vi "Main.vi"() -> ()   [LabVIEW 2020, in "Main.lvclass"]
uses:
  Main/Main.lvclass
  Coffee Shop/Coffee Shop.lvclass
  <vilib>/Asteme/Triarc Framework/Process/Process.lvclass
  <vilib>/Asteme/Triarc Framework/Application/Application.lvclass
  C:/Program Files (x86)/National Instruments/LabVIEW 2020/vi.lib/Asteme/Triarc Framework/Application/Application.lvclass
  C:/Program Files (x86)/National Instruments/LabVIEW 2020/vi.lib/Asteme/Triarc Framework/Process/Process.lvclass
  C:/Program Files (x86)/National Instruments/LabVIEW 2020/vi.lib/Asteme/Triarc Framework/Base/Base.lvclass
  C:/Program Files (x86)/National Instruments/LabVIEW 2020/vi.lib/Asteme/Triarc Framework/Error Handler Interface/Error Handler Interface.lvclass
  C:/Program Files (x86)/National Instruments/LabVIEW 2020/vi.lib/Asteme/Triarc Framework/Logging/Logging.lvclass
  C:/Users/anton/Documents/GitHub/Triarc-Examples/Coffee Shop/Coffee Shop/Coffee Shop.lvclass
panel:
  in  "Remove Customer":bool
  in  "Stop Button":bool
  in  "Remove Barista":bool
  in  "Show Barista Info":bool
  in  "Add Barista":bool
  in  "Baristas":i32(listbox)
  in  "Remove Cashier":bool
  in  "Show Cashier Info":bool
  in  "Add Cashier":bool
  in  "Cashiers":i32(listbox)
  in  "Show Customer Info":bool
  in  "Add Customer":bool
  in  "Customers":i32(listbox)
  # "Click + to add a customer actor to the system.\nClick Place Order to choose items for the customer to order.\nCustomer will wait until all items ordered are ready, then exit."
  # "Cashiers process orders into individual drink jobs and forwards those jobs to baristas.\nClick + to add a cashier actor to the system.\nClick - to remove a cashier from the system."
  # "Baristas process drink jobs and notify customers of completed drinks.\nAdd more baristas to the system by clicking +.  Pending jobs will be assigned to the next available barista.\nClick - to remove a barista from the system."
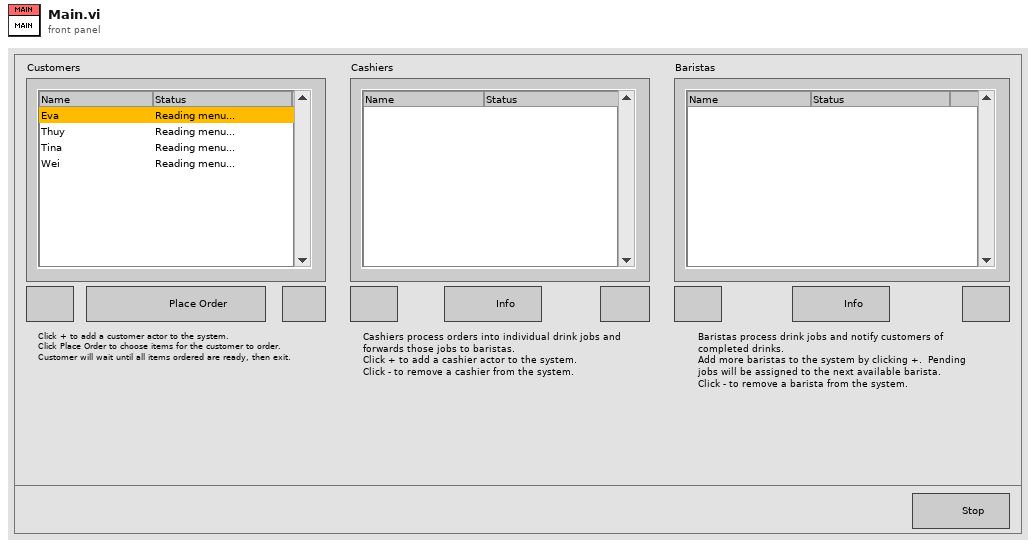
[diagram p1: front panel]
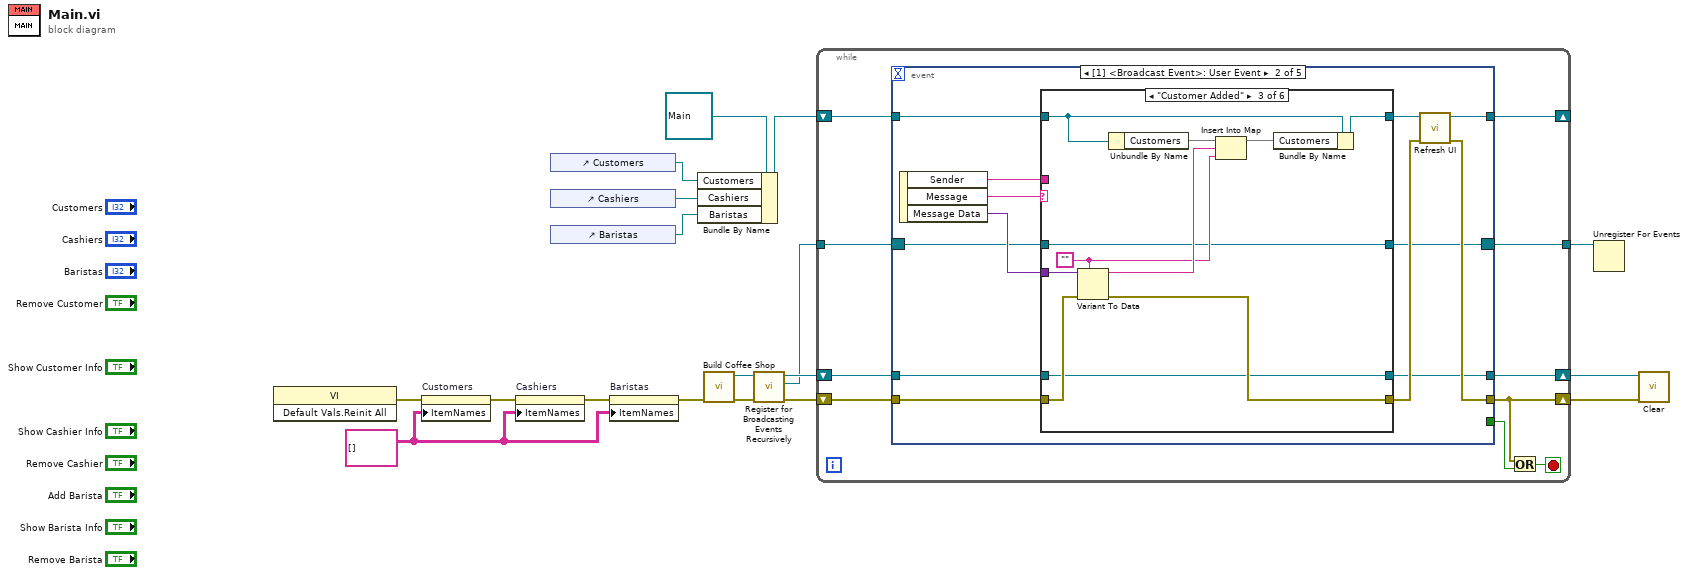
[diagram p0: block diagram]
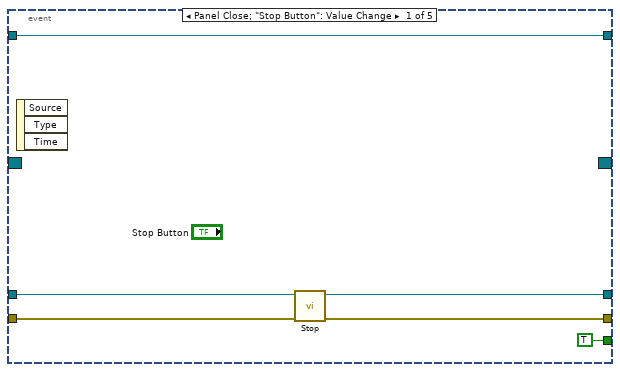
[diagram p2: hidden frame]
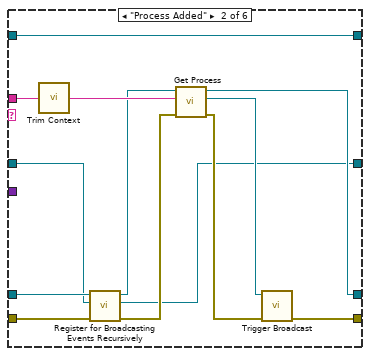
[diagram p4: hidden frame]
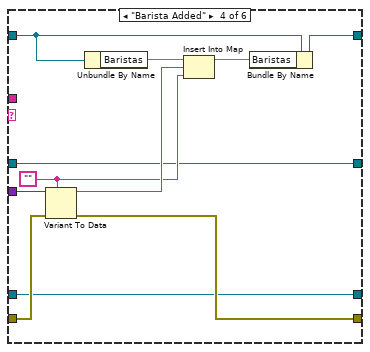
[diagram p5: hidden frame]
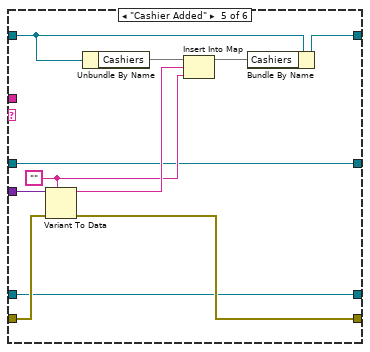
[diagram p6: hidden frame]
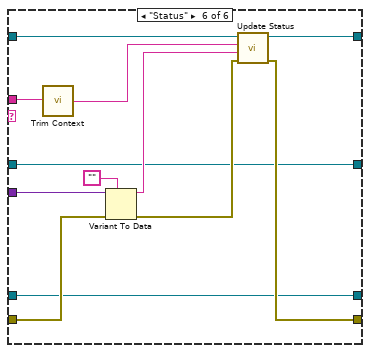
[diagram p7: hidden frame]
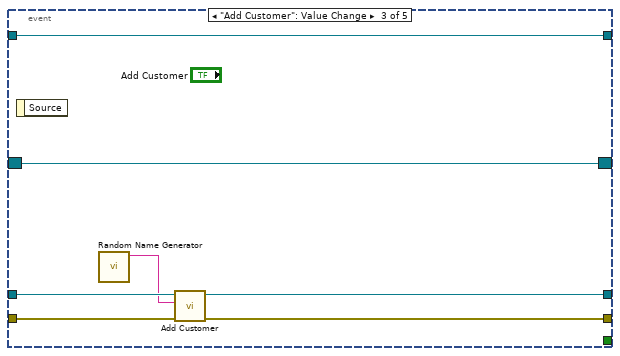
[diagram p8: hidden frame]
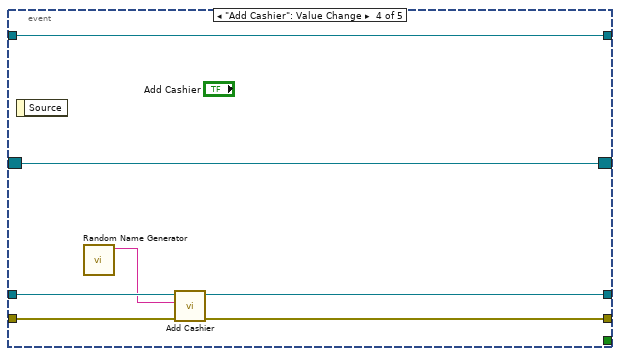
[diagram p9: hidden frame]
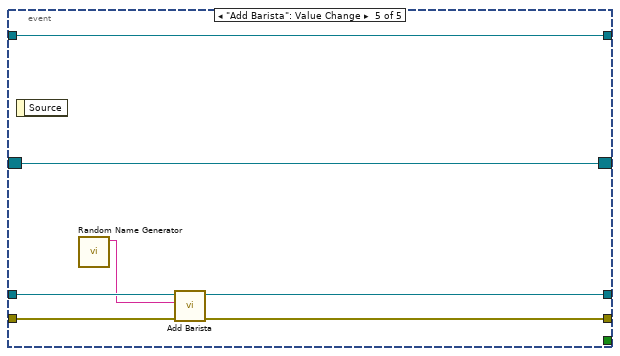
[diagram p10: hidden frame]
diagram:
  w11 = string[][] [] ("Item Names")
  n1 = invoke on="Invoke Node" class="VI" method="Default Vals.Reinit All"() -> (error out=w13:errorcluster)  [unwired: 3 in, 2 out]
  n2 = property on="Customers" class="MCListbox (strict)"(error in=w13, "ItemNames"=w11) -> (error out=w15:errorcluster)  [unwired: 1 in, 1 out]
  n3 = property on="Cashiers" class="MCListbox (strict)"(error in=w15, "ItemNames"=w11) -> (error out=w14:errorcluster)  [unwired: 1 in, 1 out]
  n4 = control-ref of="Customers"() -> (w8:refnum<vi>)
  n5 = control-ref of="Cashiers"() -> (w7:refnum<vi>)
  n6 = control-ref of="Baristas"() -> (w6:refnum<vi>)
  n7 = property on="Baristas" class="MCListbox (strict)"(error in=w14, "ItemNames"=w11) -> (error out=w12:errorcluster)  [unwired: 1 in, 1 out]
  n8 = Bundle By Name(cluster=refnum<class "Main.lvclass"> refnum ("Main.lvclass"), "Customers"=w8, "Cashiers"=w7, "Baristas"=w6) -> (w9:refnum<class "Main.lvclass">)
  n9 = call "Build Coffee Shop.vi"("error in (no error)"=w12) -> ("error out"=w4:errorcluster, "Coffee Shop Out"=w5:refnum<class "Coffee Shop.lvclass">)  [unwired: 9 in]
  n10 = call <vilib>:"Register for Broadcasting Events Recursively.vi"("error in (no error)"=w4, "Application In"=w5) -> ("error out"=w3:errorcluster, "Event Registration Refnum Out"=w1:refnum<event-registration>, "Application Out"=w2:refnum<class "Coffee Shop.lvclass">)  [unwired: 7 in]
  n11 = while {
    shift-right: [w27] -> w17
    shift-left: w3 -> [w28]
    shift-right: [w23] -> w16
    shift-left: w2 -> [w24]
    tunnel: w1 -> [w22]
    tunnel: [w21] -> w18
    shift-right: [w19] -> _
    shift-left: w9 -> [w20]
    stop <- w26 stop-if-true
    n12 = event shown="[1] <Broadcast Event>: User Event" {
      selector: w22 -> [_ w36 w112 w119 w126]
      dyn-events: [_ w35 w112 w119 w126] -> w21
      timeout: _ -> [_ _ _ _ _]
      tunnel: [w32 w42 w110 w117 w124] -> w27
      tunnel: w28 -> [w34 w44 w116 w123 w130]
      tunnel: [TRUE _ _ _ _] -> w25
      tunnel: w24 -> [w31 w37 w115 w122 w129]
      tunnel: [w30 w38 w111 w118 w125] -> w23
      tunnel: w20 -> [w29 w43 w113 w120 w127]
      tunnel: [w29 w40 w113 w120 w127] -> w19
      event Panel Close; "Stop Button": Value Change {
        n13 = event-data() -> ()  [unwired: 1 in, 3 out]
        n14 = call <vilib>:"Stop.vi"("error in (no error)"=w34, "Process In"=w31) -> ("error out"=w32:errorcluster, "Process Out"=w30:refnum<class "Coffee Shop.lvclass">)  [unwired: 7 in, 1 out]
      }
      event User Event {
        n15 = event-data() -> ("Sender"=w39:string, "Message"=w47:string, "Message Data"=w46:variant)  [unwired: 1 in]
        n16 = case shown="\"Customer Added\"" w47 {
          tunnel: w46 -> [_ _ w75 w86 w97 w102]
          tunnel: w44 -> [w51 w57 w74 w85 w96 w105]
          tunnel: [w51 w60 w73 w84 w95 w106] -> w45
          tunnel: w43 -> [w50 w64 w72 w83 w94 w107]
          tunnel: [w50 w64 w70 w81 w92 w108] -> w41
          tunnel: w39 -> [_ w63 _ _ _ w109]
          tunnel: [w49 w59 w66 w77 w88 w99] -> w38
          tunnel: w37 -> [w49 w54 w66 w77 w88 w99]
          tunnel: w36 -> [w48 w53 w65 w76 w87 w98]
          tunnel: [w48 w52 w65 w76 w87 w98] -> w35
          frame Default {
          }
          frame "Process Added" {
            n17 = call "Trim Context.vi"("Qualified Name"=w63) -> ("Name"=w61:string)
            n18 = call <vilib>:"Register for Broadcasting Events Recursively.vi"("error in (no error)"=w57, "Event Registration Refnum In"=w53, "Application In"=w54) -> ("error out"=w56:errorcluster, "Event Registration Refnum Out"=w52:refnum<event-registration>, "Application Out"=w55:refnum<class "Coffee Shop.lvclass">)  [unwired: 6 in]
            n19 = call <vilib>:"Get Process.vi"("error in (no error)"=w56, "Process Name"=w61, "Rig In"=w55) -> ("error out"=w62:errorcluster, "App Process"=w58:refnum<class "Process.lvclass">, "Rig Out"=w59:refnum<class "Coffee Shop.lvclass">)  [unwired: 6 in]
            n20 = call <vilib>:"Trigger Broadcast.vi"("error in (no error)"=w62, "Process in"=w58) -> ("error out"=w60:errorcluster)  [unwired: 8 in, 1 out]
          }
          frame "Customer Added" {
            w67 = ""
            n21 = Variant To Data(error in=w74, type=w67, Variant=w75) -> (data=w68:string, error out=w73:errorcluster)
            n22 = Unbundle By Name(w72) -> ("Customers"=w71:map{string, string})
            n23 = Insert Into Map(map in=w71, key=w68, value=w67) -> (map out=w69:map{string, string})  [unwired: 2 out]
            n24 = Bundle By Name(cluster=w72, "Customers"=w69) -> (w70:refnum<class "Main.lvclass">)
          }
          frame "Barista Added" {
            w78 = ""
            n25 = Variant To Data(error in=w85, type=w78, Variant=w86) -> (data=w79:string, error out=w84:errorcluster)
            n26 = Unbundle By Name(w83) -> ("Baristas"=w82:map{string, string})
            n27 = Insert Into Map(map in=w82, key=w79, value=w78) -> (map out=w80:map{string, string})  [unwired: 2 out]
            n28 = Bundle By Name(cluster=w83, "Baristas"=w80) -> (w81:refnum<class "Main.lvclass">)
          }
          frame "Cashier Added" {
            w89 = ""
            n29 = Variant To Data(error in=w96, type=w89, Variant=w97) -> (data=w90:string, error out=w95:errorcluster)
            n30 = Unbundle By Name(w94) -> ("Cashiers"=w93:map{string, string})
            n31 = Insert Into Map(map in=w93, key=w90, value=w89) -> (map out=w91:map{string, string})  [unwired: 2 out]
            n32 = Bundle By Name(cluster=w94, "Cashiers"=w91) -> (w92:refnum<class "Main.lvclass">)
          }
          frame "Status" {
            n33 = call "Trim Context.vi"("Qualified Name"=w109) -> ("Name"=w104:string)
            n34 = Variant To Data(error in=w105, type="", Variant=w102) -> (data=w100:string, error out=w103:errorcluster)
            n35 = call "Update Status.vi"("error in (no error)"=w103, "Status"=w100, "Name"=w104, "Main In"=w107) -> ("error out"=w106:errorcluster, "Main Out"=w108:refnum<class "Main.lvclass">)  [unwired: 6 in]
          }
        }
        n36 = call "Refresh UI.vi"("error in (no error)"=w45, "Main in"=w41) -> ("error out"=w42:errorcluster, "Main out"=w40:refnum<class "Main.lvclass">)  [unwired: 8 in]
      }
      event "Add Customer": Value Change {
        n37 = event-data() -> ()  [unwired: 1 in, 1 out]
        n38 = call "Random Name Generator.vi"() -> ("Name"=w114:string)  [unwired: 11 in]
        n39 = call "Add Customer.vi"("error in (no error)"=w116, "Name"=w114, "Coffee Shop in"=w115) -> ("error out"=w110:errorcluster, "Coffee Shop out"=w111:refnum<class "Coffee Shop.lvclass">)  [unwired: 7 in]
      }
      event "Add Cashier": Value Change {
        n40 = event-data() -> ()  [unwired: 1 in, 1 out]
        n41 = call "Random Name Generator.vi"() -> ("Name"=w121:string)  [unwired: 11 in]
        n42 = call "Add Cashier.vi"("error in (no error)"=w123, "Name"=w121, "Coffee Shop in"=w122) -> ("error out"=w117:errorcluster, "Coffee Shop out"=w118:refnum<class "Coffee Shop.lvclass">)  [unwired: 7 in]
      }
      event "Add Barista": Value Change {
        n43 = event-data() -> ()  [unwired: 1 in, 1 out]
        n44 = call "Random Name Generator.vi"() -> ("Name"=w128:string)  [unwired: 11 in]
        n45 = call "Add Barista.vi"("error in (no error)"=w130, "Name"=w128, "Coffee Shop in"=w129) -> ("error out"=w124:errorcluster, "Coffee Shop out"=w125:refnum<class "Coffee Shop.lvclass">)  [unwired: 7 in]
      }
    }
    n46 = Or(x=w27, y=w25) -> (x .or. y?=w26:bool)
  }
  n47 = Unregister For Events(event registration refnum=w18) -> ()  [unwired: 1 in, 1 out]
  n48 = call-dynamic "Clear.vi"("error in (no error)"=w17, "Application In"=w16) -> ()  [unwired: 9 in, 1 out]
